vi "写入固件.vi"(8 "错误输入":errorcluster, 11 "MB session in":refnum<class "MB_Master.lvclass">) -> (0 "error out":errorcluster, 3 "MB session out":refnum<class "MB_Master.lvclass">)   [LabVIEW 2016, in "斯坦道总磷.lvlib"]
uses:
  <vilib>/Plasmionique/MB Master/MB_Master/MB_Master.lvclass
  <vilib>/NI/Progress Bar/Controls/Update Bar Actions.ctl
  <vilib>/NI/Progress Bar/Controls/Progress Bar Properties.ctl
  <vilib>/Plasmionique/MB Master/MB_Master_Serial/MB_Master_Serial.lvclass
  C:/Program Files (x86)/National Instruments/LabVIEW 2016/vi.lib/Plasmionique/MB Master/MB_Master/MB_Master.lvclass
  <vilib>/Plasmionique/MB Master/MB Master.lvlib
  <vilib>/NI/Progress Bar/Progress Bar.lvlib
panel:
  in  "引用选择":enum16{"MB引用", "自建引用"}(ring)
  in  "VISA Resource":refnum<visa-resource-name>
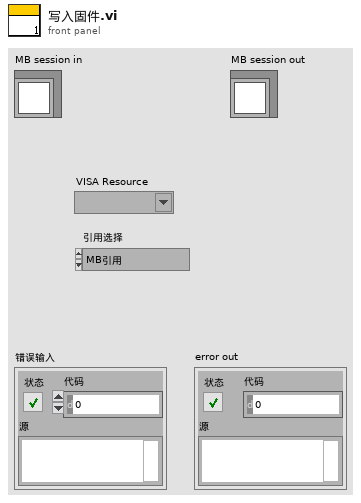
[diagram p1: front panel]
types:
  T1 = enum16{"open", "replace", "create", "open or create", "replace or create", "replace or create with confirmation"}
  T2 = enum16{"big-endian, network order", "native, host order", "little-endian"}
  T3 = typedef "Progress Bar.lvlib/Update Bar Actions.ctl" = enum16{"Add To Existing", "Set to Value"}
  T4 = cluster{"baud rate (bps)":u32, "stop bits":u16, "parity":u16, "flow control":u16, "timeout":u32, "retries":i32}
  T5 = typedef "Progress Bar.lvlib/Progress Bar Properties.ctl" = cluster{"Background Color":u32, "Installer Title":string, "Title Color":u32, "Action Text":string, "Text Color":u32, "Slider Value":u8, "Bar Color":u32, "Timeout":i32}
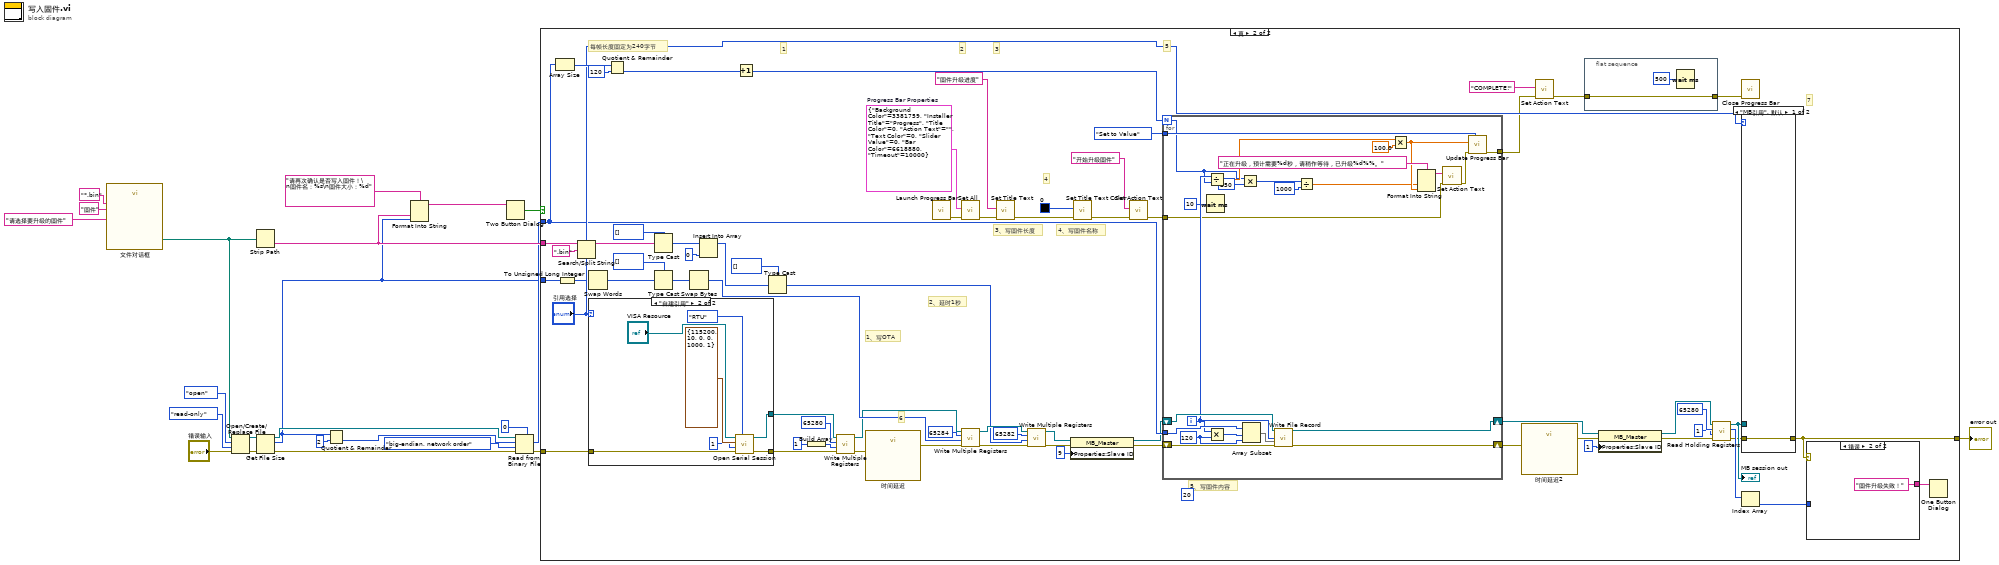
[diagram p0: block diagram]
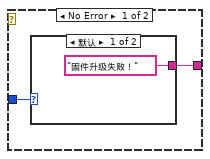
[diagram p3: hidden frame]
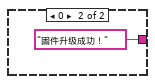
[diagram p4: hidden frame]
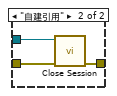
[diagram p5: hidden frame]
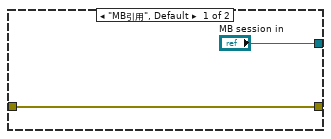
[diagram p6: hidden frame]
diagram:
  n1 = call "文件对话框"("prompt"="请选择要升级的固件", "pattern (all files)"="*.bin", "pattern label"="固件") -> ("selected path"=w10:path)  [unwired: 9 in, 3 out]
  n2 = Open/Create/Replace File(file path (use dialog)=w10, error in="错误输入", operation (0:open)=T1."open" ("操作(0:open)"), access (0:read/write)=enum16{"read/write", "read-only", "write-only"}."read-only" ("权限(0:read/write)")) -> (refnum out=w9:refnum<file>, error out=w7:errorcluster)  [unwired: 2 in, 1 out]
  n3 = Strip Path(path=w10) -> (name=w18:string)  [unwired: 1 out]
  n4 = Get File Size(file=w9, error in=w7) -> (refnum out=w8:refnum<file>, size (in bytes)=w2:i64, 0:w6:errorcluster)
  n5 = Quotient & Remainder(x=w2, y=i64 2) -> (floor(x/y)=w4:i64)  [unwired: 1 out]
  n6 = Format Into String(format string="请再次确认是否写入固件！\n固件名：%s\n固件大小：%d" ("格式字符串"), w18, w2) -> (resulting string=w17:string)  [unwired: 2 in, 1 out]
  n7 = Two Button Dialog(message=w17) -> (T button?=w16:bool)  [unwired: 2 in]
  n8 = Read from Binary File(5:u16 0, 8:w6, 9:T2."big-endian, network order" ("字节顺序(0:big-endian, network order)"), 10:w4, 11:w8) -> (0:w15:errorcluster, 2:w3:u16[])  [unwired: 1 in, 2 out]
  n9 = case shown="真" w16 {
    tunnel: w3 -> [_ w55]
    tunnel: w18 -> [_ w71]
    tunnel: w15 -> [w24 w74]
    tunnel: [w24 w42] -> w13
    tunnel: w2 -> [_ w57]
    frame False {
    }
    frame True {
      w39 = T5 {"Background Color"=3381759, "Installer Title"="Progress", "Title Color"=0, "Action Text"="", "Text Color"=0, "Slider Value"=0, "Bar Color"=6618880, "Timeout"=10000}  # Progress Bar Properties
      (unwired) 20 ("Value")
      # "7"
      # "6"
      # "5"
      # "4"
      # "3"
      # "2"
      # "1"
      # "每帧长度固定为240字节"
      # "5、写固件内容"
      # "4、写固件名称"
      # "3、写固件长度"
      # "2、延时1秒"
      # "1、写OTA"
      n10 = Array Size(array=w55) -> (size(s)=w90:i32)
      n11 = To Unsigned Long Integer(number=w57) -> (unsigned 32bit integer=w49:u32)
      n12 = Search/Split String(string=w71, search string/char (-)=".bin" ("搜索字符串/字符(-)")) -> (substring before match=w69:string)  [unwired: 1 in, 2 out]
      n13 = Swap Words(1:w49) -> (0:w48:u32)
      n14 = case shown="\"自建引用\"" "引用选择" {
        tunnel: ["MB session in" w110] -> w75
        tunnel: w74 -> [w104 w109]
        tunnel: [w104 w108] -> w73
        frame "MB引用", Default {
        }
        frame "自建引用" {
          n15 = call <vilib>:"Open Serial Session.vi"("Mode (RTU)"=enum16{"RTU", "ASCII"}."RTU", "Error in"=w109, "Slave ID"=u8 1, "Serial Config"=T4 {"baud rate (bps)"=115200, "stop bits"=10, "parity"=0, "flow control"=0, "timeout"=1000, "retries"=1}, "VISA Resource"="VISA Resource") -> ("Error out"=w108:errorcluster, "MB_Serial session"=w110:refnum<class "MB_Master_Serial.lvclass">)  [unwired: 5 in]
        }
      }
      n16 = Quotient & Remainder(x=w90, y=120) -> (floor(x/y)=w91:i32)  [unwired: 1 out]
      n17 = Type Cast(type=u8[] [], x=w69) -> (*(type *) &x=w78:u8[])
      n18 = Type Cast(type=u16[] [], x=w48) -> (*(type *) &x=w84:u16[])
      n19 = Swap Bytes(anything=w84) -> (byte swapped=w83:u16[])
      n20 = Insert Into Array(array=w78, new element=u8 0 ("新元素/子数组")) -> (w68:u8[])  [unwired: 1 in]
      n21 = Increment(x=w91) -> (x+1=w56:i32)
      n22 = Type Cast(type=u16[] [], x=w68) -> (*(type *) &x=w67:u16[])
      n23 = Build Array(u16 1 ("value")) -> (w76:u16[])
      n24 = call <vilib>:"Write Multiple Registers.vi"("error in (no error)"=w73, "values"=w76, "starting address"=u16 65280, "MB session in"=w75) -> ("error out"=w86:errorcluster, "MB session out"=w60:refnum<class "MB_Master.lvclass">)  [unwired: 6 in]
      n25 = call "时间延迟"("error in (no error)"=w86) -> ("error out"=w61:errorcluster)  [unwired: 10 in]
      n26 = call <vilib>:"Launch Progress Bar.vi"() -> ("error out"=w38:errorcluster)  [unwired: 10 in, 1 out]
      n27 = call <vilib>:"Set All.vi"("error in (no error)"=w38, "Progress Bar Properties (Default)"=w39) -> ("error out"=w32:errorcluster)  [unwired: 9 in]
      n28 = call <vilib>:"Write Multiple Registers.vi"("error in (no error)"=w61, "values"=w83, "starting address"=u16 65284, "MB session in"=w60) -> ("error out"=w81:errorcluster, "MB session out"=w82:refnum<class "MB_Master.lvclass">)  [unwired: 6 in]
      n29 = call <vilib>:"Set Title Text.vi"("error in (no error)"=w32, "Installer Title"="固件升级进度") -> ("error out"=w30:errorcluster)  [unwired: 9 in]
      n30 = call <vilib>:"Write Multiple Registers.vi"("error in (no error)"=w81, "values"=w67, "starting address"=u16 65282, "MB session in"=w82) -> ("error out"=w51:errorcluster, "MB session out"=w54:refnum<class "MB_Master.lvclass">)  [unwired: 6 in]
      n31 = property class="MB_Master"(reference=w54, error in=w51, "Properties:Slave ID"=u8 9 ("Slave ID")) -> (reference out=w52:refnum<class "MB_Master.lvclass">, error out=w50:errorcluster)
      n32 = call <vilib>:"Set Title Text Color.vi"("error in (no error)"=w30, "Color Box"=u32 0) -> ("error out"=w33:errorcluster)  [unwired: 9 in]
      n33 = call <vilib>:"Set Action Text.vi"("error in (no error)"=w33, "Action Text"="开始升级固件") -> ("error out"=w27:errorcluster)  [unwired: 9 in]
      n34 = for {
        N: w56 -> [w113]
        shift-right: [w133] -> w47
        shift-left: w52 -> [w135]
        shift-right: [w131] -> w45
        shift-left: w50 -> [w134]
        tunnel: w55 -> [w130]
        tunnel: Update_Bar_Actions."Set to Value" ("Action") -> [w125]
        tunnel: w27 -> [w123]
        tunnel: [w124] -> w26
        i -> [w128]
        w127 = 120 ("长度")
        n35 = Wait (ms)(milliseconds to wait=u32 10) -> ()  [unwired: 1 out]
        n36 = Divide(x=w128, y=w113) -> (x/y=w119:dbl)
        n37 = Multiply(x=w128, y=w127) -> (x*y=w126:i32)
        n38 = Multiply(x=w113, y=250) -> (x*y=w117:i32)
        n39 = Array Subset(array=w130, index=w126, length=w127) -> (w129:u16[])
        n40 = call "Write File Record.vi"("MB session in"=w135, "Record Number"=w128, "values"=w129, "error in (no error)"=w134) -> ("MB session out"=w133:refnum<class "MB_Master.lvclass">, "error out"=w131:errorcluster)  [unwired: 10 in]
        n41 = Divide(x=w117, y=u32 1000) -> (x/y=w114:dbl)
        n42 = Multiply(x=w119, y=100.0) -> (x*y=w115:dbl)
        n43 = Format Into String(format string="正在升级，预计需要%d秒，请稍作等待，已升级%d%%。" ("格式字符串"), w114, w115) -> (resulting string=w120:string)  [unwired: 2 in, 1 out]
        n44 = call <vilib>:"Set Action Text.vi"("error in (no error)"=w123, "Action Text"=w120) -> ("error out"=w122:errorcluster)  [unwired: 9 in]
        n45 = call <vilib>:"Update Progress Bar.vi"("Action"=w125, "error in (no error)"=w122, "Value"=w115) -> ("error out"=w124:errorcluster)  [unwired: 8 in]
      }
      n46 = call "时间延迟2"("error in (no error)"=w45) -> ("error out"=w25:errorcluster)  [unwired: 10 in]
      n47 = call <vilib>:"Set Action Text.vi"("error in (no error)"=w26, "Action Text"="COMPLETE!") -> ("error out"=w35:errorcluster)  [unwired: 9 in]
      n48 = flat-sequence {
        tunnel: w35 -> [w92]
        tunnel: [w92] -> w37
        frame #0 {
          n49 = Wait (ms)(milliseconds to wait=u32 500) -> ()  [unwired: 1 out]
        }
      }
      n50 = property class="MB_Master"(reference=w47, error in=w25, "Properties:Slave ID"=u8 1 ("Slave ID")) -> (reference out=w46:refnum<class "MB_Master.lvclass">, error out=w44:errorcluster)
      n51 = call <vilib>:"Read Holding Registers.vi"("error in (no error)"=w44, "quantity"=u16 1, "starting address"=u16 65280, "MB session in"=w46) -> ("error out"=w58:errorcluster, "Registers"=w62:u16[], "MB session out"=w59:refnum<class "MB_Master.lvclass">)  [unwired: 5 in]
      "MB session out" <- w59
      n52 = call <vilib>:"Close Progress Bar.vi"("error in (no error)"=w37) -> ()  [unwired: 9 in, 2 out]
      n53 = case shown="\"MB引用\", 默认" "引用选择" {
        tunnel: w59 -> [_ w102]
        tunnel: w58 -> [w99 w101]
        tunnel: [w99 w100] -> w42
        frame "MB引用", Default {
        }
        frame "自建引用" {
          n54 = call-dynamic "Close Session.vi"("error in (no error)"=w101, "MB session in"=w102) -> ("error out"=w100:errorcluster)  [unwired: 9 in]
        }
      }
      n55 = Index Array(array=w62) -> (element=w41:u16)  [unwired: 1 in]
      n56 = case shown="错误" w42 {
        tunnel: w41 -> [w95 _]
        tunnel: [w94 "固件升级失败！"] -> w40
        frame No Error {
          n57 = case shown="默认" w95 {
            tunnel: ["固件升级失败！" "固件升级成功！"] -> w94
            frame Default {
            }
            frame 0 {
            }
          }
        }
        frame Error {
        }
      }
      n58 = One Button Dialog(message=w40) -> ()  [unwired: 1 in, 1 out]
    }
  }
  "error out" <- w13
